vi "Initialization VI.vi"(8 "error in (no error)":errorcluster, 10 "Custom XML":string, 11 "Device Item Ref in":T1 format="%.0x") -> (0 "error out":errorcluster, 3 "Device Item Ref out":T1 format="%.0x")   [LabVIEW 2015, in "Protection and Counter Addon System Explorer.lvlib"]
uses:
  Protection and Counter Addon System Explorer.lvlib
  <vilib>/NI Veristand/Custom Device API/Custom Device Item Ref.ctl
  <vilib>/NI Veristand/Custom Device API/Custom Device Channel.ctl
  <vilib>/NI Veristand/Custom Device API/Custom Device Channel Type.ctl
  Shared/SubVIs/GUID Lookup.vi
  <vilib>/NI VeriStand/Custom Device API/Custom Device API.lvlib
  Shared/Protection and Counter Addon Shared.lvlib
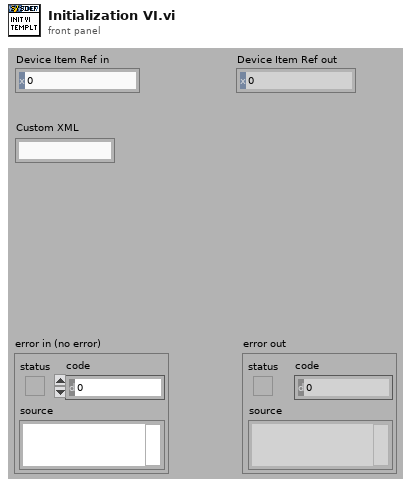
[diagram p1: front panel]
types:
  T1 = typedef "Custom Device API.lvlib/Custom Device Item Ref.ctl" = u64
  T2 = typedef "Custom Device API.lvlib/Custom Device Channel.ctl" = cluster{"Type":T3, "Units":string, "Default Value":dbl, "Faultable":bool, "Scalable":bool}
  T3 = typedef "Custom Device API.lvlib/Custom Device Channel Type.ctl" = enum16{"Input", "Output"}
  T4 = typedef "Protection and Counter Addon Shared.lvlib/XNET Settings.ctl" = cluster{"Database":refnum<k21>, "Cluster":refnum<k21>, "Port":string, "Baud rate [Bd]":u64, "Termination":u32, "CAN I/O Mode":u32, "FD Baud rate [Bd]":u64, "Priority":i32, "Use Legacy":bool}
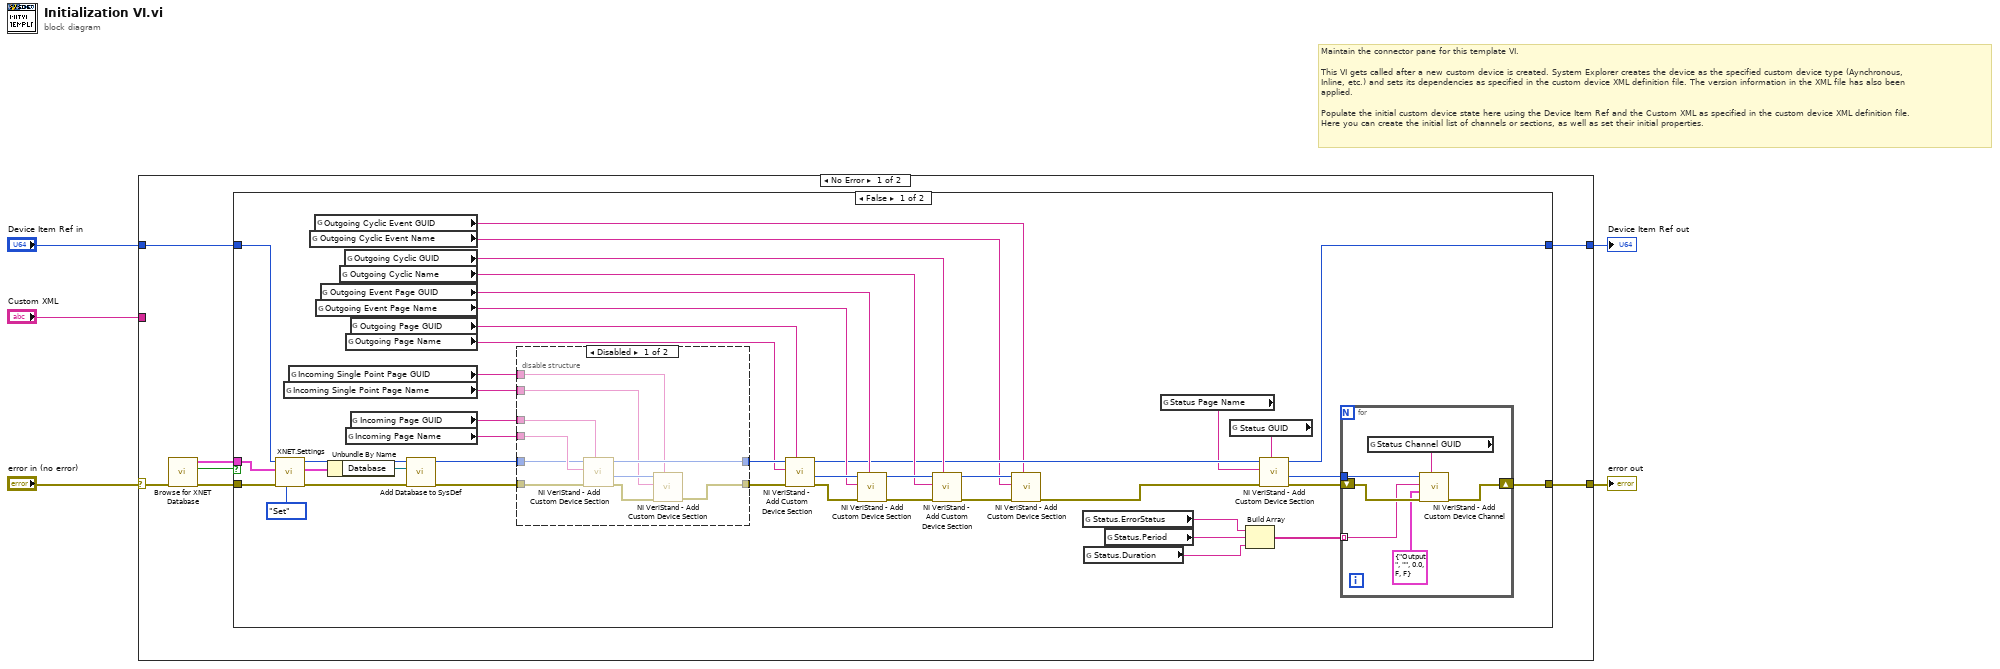
[diagram p0: block diagram]
diagram:
  # "Maintain the connector pane for this template VI.\n\nThis VI gets called after a new custom device is created. System Explorer creates the device as the specified custom device type (Aynchronous, Inline, etc.) and sets its dependencies as specified in the custom device XML definition file. The version information in the XML file has also been applied.\n\nPopulate the initial custom device state here using the Device Item Ref and the Custom XML as specified in the custom device XML definition file. Here you can create the initial list of channels or sections, as well as set their initial properties."
  n1 = case shown="No Error" "error in (no error)" {
    selector: "error in (no error)" -> [w10 w76]
    tunnel: [w12 w76] -> w5
    tunnel: [w11 w75] -> w3
    tunnel: "Device Item Ref in" -> [w8 w75]
    tunnel: "Custom XML" -> [_ _]
    frame No Error {
      n2 = call "Browse for XNET Database.vi"("error in (no error)"=w10) -> ("error out"=w9:errorcluster, "Cancel Out"=w7:bool, "XNET Settings"=w6:T4)  [unwired: 8 in]
      n3 = case shown="False" w7 {
        tunnel: [w24 w74] -> w12
        tunnel: [w25 w73] -> w11
        tunnel: w9 -> [w47 w74]
        tunnel: w8 -> [w45 w73]
        tunnel: w6 -> [w43 _]
        frame False {
          n4 = call "XNET.Settings.vi"("Action"=enum8{"Get", "Set"}."Set", "error in (no error)"=w47, "XNET Settings"=w43, "Parent Ref in"=w45) -> ("error out"=w46:errorcluster, "XNET Settings"=w42:T4, "Item Ref out"=w44:T1)  [unwired: 5 in]
          n5 = global read "GUID Lookup.vi" "Incoming Single Point Page Name"() -> (w29:string)
          n6 = global read "GUID Lookup.vi" "Incoming Single Point Page GUID"() -> (w30:string)
          n7 = global read "GUID Lookup.vi" "Outgoing Cyclic Event Name"() -> (w13:string)
          n8 = global read "GUID Lookup.vi" "Outgoing Cyclic Event GUID"() -> (w14:string)
          n9 = global read "GUID Lookup.vi" "Outgoing Event Page Name"() -> (w34:string)
          n10 = global read "GUID Lookup.vi" "Outgoing Event Page GUID"() -> (w35:string)
          n11 = Unbundle By Name(w42) -> ("Database"=w41:refnum<k21>)
          n12 = global read "GUID Lookup.vi" "Outgoing Cyclic Name"() -> (w32:string)
          n13 = global read "GUID Lookup.vi" "Outgoing Cyclic GUID"() -> (w33:string)
          n14 = global read "GUID Lookup.vi" "Outgoing Page Name"() -> (w51:string)
          n15 = global read "GUID Lookup.vi" "Incoming Page Name"() -> (w50:string)
          n16 = global read "GUID Lookup.vi" "Outgoing Page GUID"() -> (w52:string)
          n17 = global read "GUID Lookup.vi" "Incoming Page GUID"() -> (w54:string)
          n18 = call "Add Database to SysDef.vi"("error in"=w46, "DB Alias"=w41, "Item Ref in"=w44) -> ("error out"=w49:errorcluster, "Item Ref out"=w48:T1)  [unwired: 7 in]
          n19 = disable-structure shown="Disabled" {
            disable-tunnel: w54 -> [w70 _]
            disable-tunnel: [w69 w71] -> w53
            disable-tunnel: w50 -> [w68 _]
            disable-tunnel: w49 -> [w67 w72]
            disable-tunnel: w48 -> [w66 w71]
            disable-tunnel: [w63 w72] -> w31
            disable-tunnel: w30 -> [w62 _]
            disable-tunnel: w29 -> [w61 _]
            frame Disabled {
              n20 = call <vilib>:"NI VeriStand - Add Custom Device Section.vi"("GUID (Default Section)"=w70, "error in (no error)"=w67, "Section Name"=w68, "Parent Ref in"=w66) -> ("error out"=w64:errorcluster, "Section Ptr"=w65:T1, "Parent Ref out"=w69:T1)  [unwired: 4 in, 1 out]
              n21 = call <vilib>:"NI VeriStand - Add Custom Device Section.vi"("GUID (Default Section)"=w62, "error in (no error)"=w64, "Section Name"=w61, "Parent Ref in"=w65) -> ("error out"=w63:errorcluster)  [unwired: 4 in, 3 out]
            }
            frame Enabled {
            }
          }
          n22 = call <vilib>:"NI VeriStand - Add Custom Device Section.vi"("GUID (Default Section)"=w52, "error in (no error)"=w31, "Section Name"=w51, "Parent Ref in"=w53) -> ("error out"=w37:errorcluster, "Section Ptr"=w39:T1, "Parent Ref out"=w26:T1)  [unwired: 4 in, 1 out]
          n23 = call <vilib>:"NI VeriStand - Add Custom Device Section.vi"("GUID (Default Section)"=w35, "error in (no error)"=w37, "Section Name"=w34, "Parent Ref in"=w39) -> ("error out"=w38:errorcluster, "Parent Ref out"=w36:T1)  [unwired: 4 in, 2 out]
          n24 = call <vilib>:"NI VeriStand - Add Custom Device Section.vi"("GUID (Default Section)"=w33, "error in (no error)"=w38, "Section Name"=w32, "Parent Ref in"=w36) -> ("error out"=w16:errorcluster, "Parent Ref out"=w17:T1)  [unwired: 4 in, 2 out]
          n25 = call <vilib>:"NI VeriStand - Add Custom Device Section.vi"("GUID (Default Section)"=w14, "error in (no error)"=w16, "Section Name"=w13, "Parent Ref in"=w17) -> ("error out"=w15:errorcluster)  [unwired: 4 in, 3 out]
          n26 = global read "GUID Lookup.vi" "Status.ErrorStatus"() -> (w23:string)
          n27 = global read "GUID Lookup.vi" "Status.Duration"() -> (w21:string)
          n28 = global read "GUID Lookup.vi" "Status.Period"() -> (w22:string)
          n29 = global read "GUID Lookup.vi" "Status Page Name"() -> (w18:string)
          n30 = global read "GUID Lookup.vi" "Status GUID"() -> (w19:string)
          n31 = Build Array(w23, w22, w21) -> (w20:string[])
          n32 = call <vilib>:"NI VeriStand - Add Custom Device Section.vi"("GUID (Default Section)"=w19, "error in (no error)"=w15, "Section Name"=w18, "Parent Ref in"=w26) -> ("error out"=w27:errorcluster, "Section Ptr"=w28:T1, "Parent Ref out"=w25:T1)  [unwired: 4 in, 1 out]
          n33 = for {
            tunnel: w28 -> [w60]
            shift-right: [w58] -> w24
            shift-left: w27 -> [w59]
            tunnel: w20 -> [w55] mode=indexing
            n34 = global read "GUID Lookup.vi" "Status Channel GUID"() -> (w57:string)
            n35 = call <vilib>:"NI VeriStand - Add Custom Device Channel.vi"("GUID (Default Channel)"=w57, "error in (no error)"=w59, "Channel"=T2 {"Type"=enum."Output", "Units"="", "Default Value"=0.0, "Faultable"=FALSE, "Scalable"=FALSE}, "Channel Name"=w55, "Parent Ref in"=w60) -> ("error out"=w58:errorcluster)  [unwired: 3 in, 3 out]
          }
        }
        frame True {
        }
      }
    }
    frame Error {
    }
  }
  "error out" <- w5
  "Device Item Ref out" <- w3
